vi "U3 Multiple IO Example.vi"() -> ()   [LabVIEW 2021]
panel:
  out "FIO5":bool
  out "FIO4":bool
  out "AIN3":dbl format="%.6f"
  out "AIN2":dbl format="%.6f"
  out "AIN1":dbl format="%.6f"
  out "AIN0":dbl format="%.6f"
  in  "FIO7":bool
  in  "FIO6":bool
  in  "DAC0":dbl format="%.4f"
  out "Error Message":string
  out "error out":errorcluster
  # "Outputs DAC0 and FIO6-FIO7.  Aquires AIN0-AIN3 and FIO4-FIO5.  This example\ndoes the proper pin configuration also.  Uses USB on the first found U3."
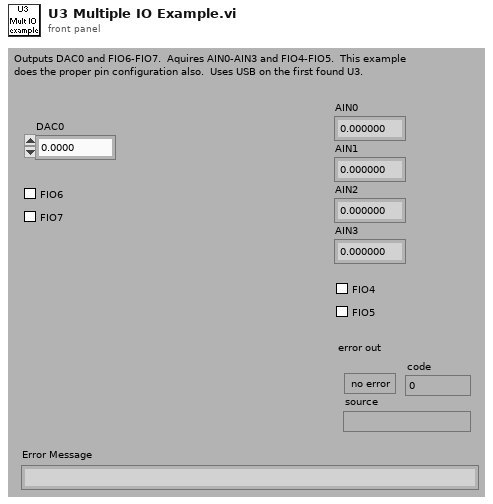
[diagram p1: front panel]
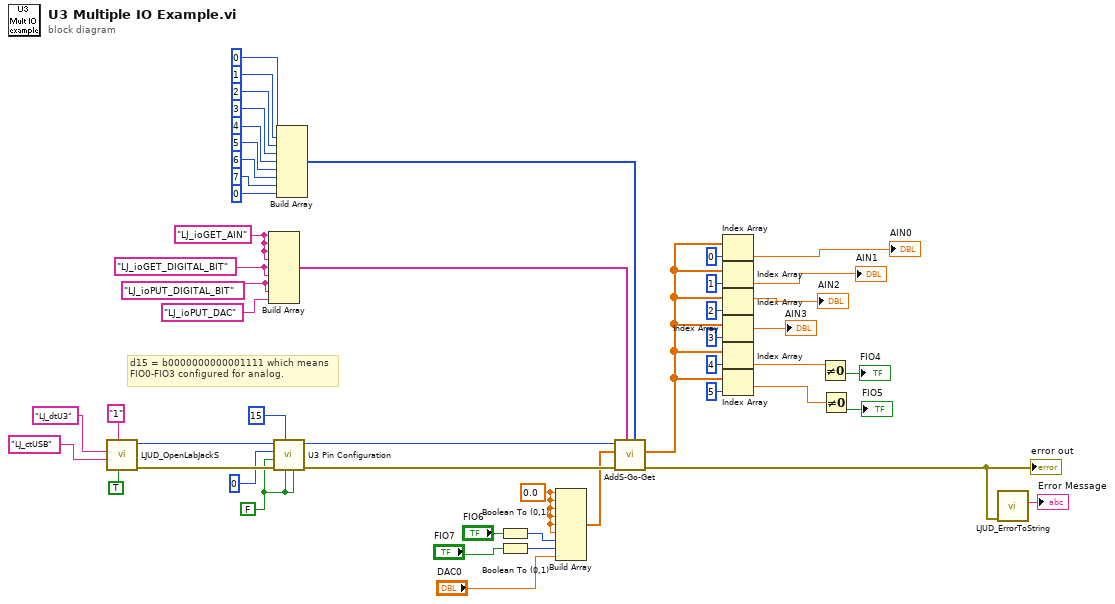
[diagram p0: block diagram]
diagram:
  w23 = 0.0 ("Input Element")
  w24 = FALSE ("Enable DAC1")
  w47 = "LJ_ioPUT_DIGITAL_BIT" ("IOType")
  w49 = "LJ_ioGET_AIN" ("IOType")
  w48 = "LJ_ioGET_DIGITAL_BIT" ("IOType")
  # "d15 = b0000000000001111 which means\nFIO0-FIO3 configured for analog."
  n1 = call "LJUD_OpenLabJackS.vi"("FirstFound"=TRUE, "Address"="1", "ConnectionType"="LJ_ctUSB", "DeviceType"="LJ_dtU3") -> ("error out"=w29:errorcluster, "Handle"=w27:i32)  [unwired: 5 in, 1 out]
  n2 = Build Array(w49, w49, w49, w49, w48, w48, w47, w47, "LJ_ioPUT_DAC" ("IOType")) -> (w46:string[])
  n3 = call "U3 Pin Configuration.vi"("Enable Counter1"=w24, "Enable Counter0"=w24, "FIO/EIO Analog Enable"=15, "error in"=w29, "Enable DAC1"=w24, "Number of Timers Enabled"=u8 0, "Handle In"=w27) -> ("error out"=w30:errorcluster, "Handle Out"=w28:i32)  [unwired: 3 in]
  n4 = Build Array(0, 1, 2, 3, 4, 5, 6, 7, 0) -> (w45:i32[])
  n5 = Boolean To (0,1)(Boolean="FIO6") -> (0, 1=w22:i16)
  n6 = Boolean To (0,1)(Boolean="FIO7") -> (0, 1=w21:i16)
  n7 = Build Array(w23, w23, w23, w23, w23, w23, w22, w21, "DAC0") -> (w20:dbl[])
  n8 = call "AddS-Go-Get.vi"("Channels"=w45, "IOTypes"=w46, "error in"=w30, "Values Write"=w20, "Handle In"=w28) -> ("error out"=w1:errorcluster, "Values Read"=w14:dbl[])  [unwired: 4 in, 1 out]
  "error out" <- w1
  n9 = Index Array(array=w14, index=0 ("Index")) -> (element=→"AIN0":dbl)
  n10 = Index Array(array=w14, index=1 ("Index")) -> (element=→"AIN1":dbl)
  n11 = Index Array(array=w14, index=2 ("Index")) -> (element=→"AIN2":dbl)
  n12 = Index Array(array=w14, index=3 ("Index")) -> (element=→"AIN3":dbl)
  n13 = Index Array(array=w14, index=4 ("Index")) -> (element=w12:dbl)
  n14 = Index Array(array=w14, index=5 ("Index")) -> (element=w11:dbl)
  n15 = Not Equal To 0?(x=w12) -> (x != 0?=→"FIO4":bool)
  n16 = Not Equal To 0?(x=w11) -> (x != 0?=→"FIO5":bool)
  n17 = call "LJUD_ErrorToString.vi"("error in"=w1) -> ("String"=→"Error Message":string)  [unwired: 10 in]
